vi "ODMR sweep ACCES DAC WF control.vi"(5 "leveling file":path=path "C:/Users/Ouyang Group/Documents/Data/8-26-16/Windfreak plus switches and amp power calibration high res", 6 "p (dbm)":dbl=-4.0, 7 "leveling":bool=TRUE, 8 "Save?":bool, 9 "file path (dialog if empty)":path, 10 "Freq Sweep Cluster":T1={"GPIB address 2"="19", "resolution (10 Hz:2) 2"=2, "band (1-26.5:2) 2"=2, "Freq max"=3000000000.0, "Start Freq"=2700000000.0, "Freq Step"=10000000.0, "rate"=100.0, "samples per channel"=200} {"rate" format="%0.2f"; "resolution (10 Hz:2) 2" items=["0.1 Hz", "1 Hz", "10 Hz", "100 Hz", "1 KHz", "10 KHz", "100 KHz", "1 MHz", "10 MHz", "100 MHz", "1 GHz"]}, 11 "Dot Tracking Cluster":T2={"RS232 settings"={"Portnumber"=12, "Baudrate"=5}, "X Parameters"={"Number of X Steps"=200, "Max X (V)"=2.0, "Min X (V)"=-2.0}, "Y Parameters"={"Number of Y Steps"=200, "Max Y (V)"=2.0, "Min Y (V)"=-2.0}, "X Pos"=97.0, "Y Pos"=112.0, "Z Pos"=52.78, "Tracking interval"=150.0} {"RS232 settings"."Portnumber" items=["COM1", "COM2", "COM3", "COM4", "COM5", "COM6", "COM7", "COM8", "COM9", "COM10", "COM11", "COM12", "COM13", "COM14", "COM15", "COM16", "COM17", "COM18", "COM19", "COM20", "COM21", "COM22", "COM23", "COM24", "COM25", "COM26", "COM27", "COM28", "COM29", "COM30"]; "RS232 settings"."Baudrate" items=["9600", "14400", "19200", "38400", "57600", "115200"]}) -> (0 "Z Position":dbl=31.0, 1 "Y Position":dbl=62.0, 2 "X Position":dbl=97.0, 3 "XY Graph":cluster{"Y":dbl[], "Y":dbl[]}[](graph), 4 "appended array":ext[][](array[numeric]))   [LabVIEW 2012]
uses:
  <vilib>/DAQmx/read.llb/DAQmx Read (Counter 1D DBL 1Chan NSamp).vi
  <vilib>/DAQmx/create/channels.llb/DAQmx Create Channel (CI-Count Edges).vi
  <vilib>/DAQmx/configure/timing.llb/DAQmx Timing (Sample Clock).vi
  <vilib>/DAQmx/miscellaneous.llb/DAQmx Fill In Error Info.vi
  <vilib>/Utility/file.llb/Write To Spreadsheet File (DBL).vi
  <resource>/objmgr/daqmx.rc
panel:
  out "COM Error":bool
  out "Level":bool
  out "power":dbl
  out "Frequency":dbl
  in  "stop":bool
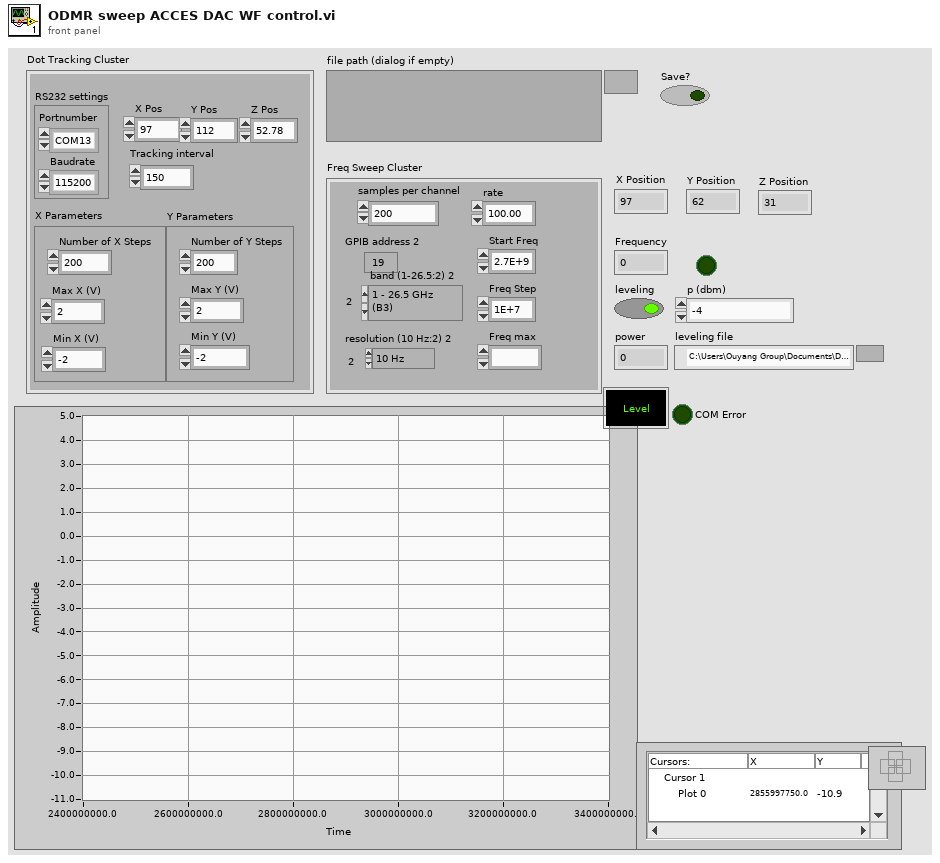
[diagram p1: front panel]
types:
  T1 = cluster{"GPIB address 2":string, "resolution (10 Hz:2) 2":i32, "band (1-26.5:2) 2":i32, "Freq max":ext, "Start Freq":dbl, "Freq Step":dbl, "rate":dbl, "samples per channel":i32}
  T2 = cluster{"RS232 settings":cluster{"Portnumber":i32, "Baudrate":u16}, "X Parameters":cluster{"Number of X Steps":i32, "Max X (V)":dbl, "Min X (V)":dbl}, "Y Parameters":cluster{"Number of Y Steps":i32, "Max Y (V)":dbl, "Min Y (V)":dbl}, "X Pos":dbl, "Y Pos":dbl, "Z Pos":dbl, "Tracking interval":dbl}
  T3 = cluster{"Number of X Steps":i32, "Max X (V)":dbl, "Min X (V)":dbl}
  T4 = cluster{"Number of Y Steps":i32, "Max Y (V)":dbl, "Min Y (V)":dbl}
  T5 = cluster{"source lock":bool, "lock frequency (Hz)":ext, "coarse tune":bool}
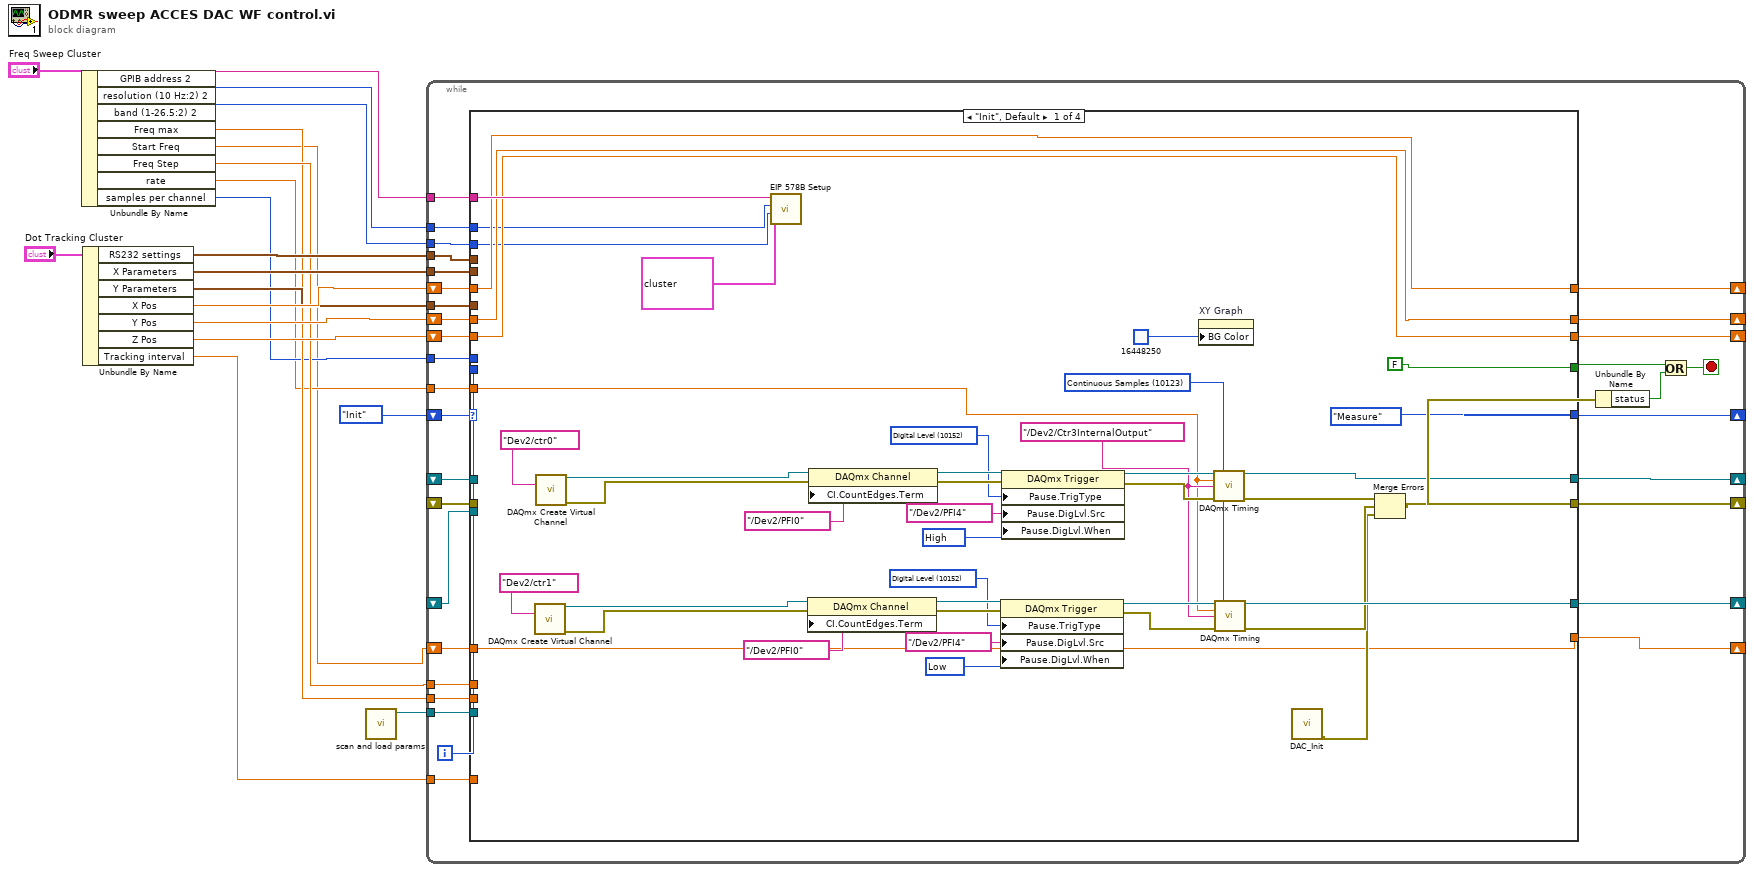
[diagram p0: block diagram]
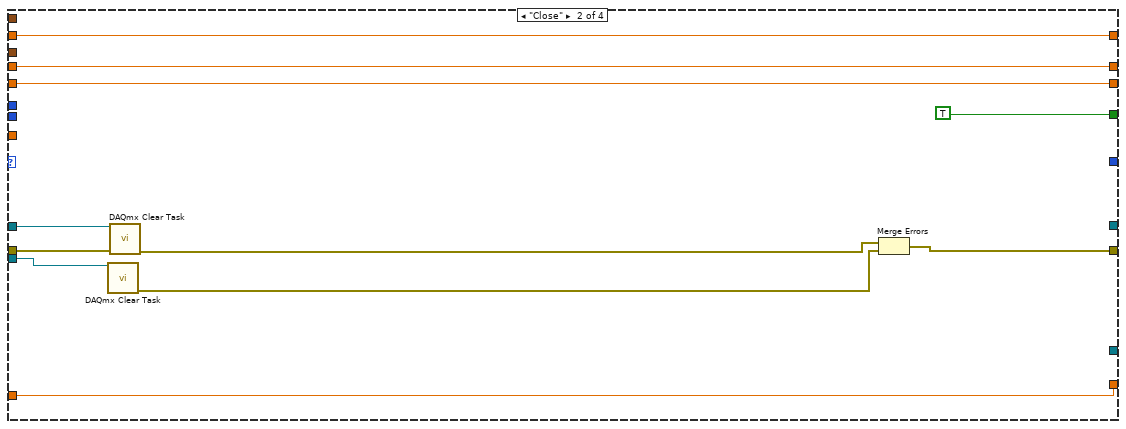
[diagram p2: hidden frame]
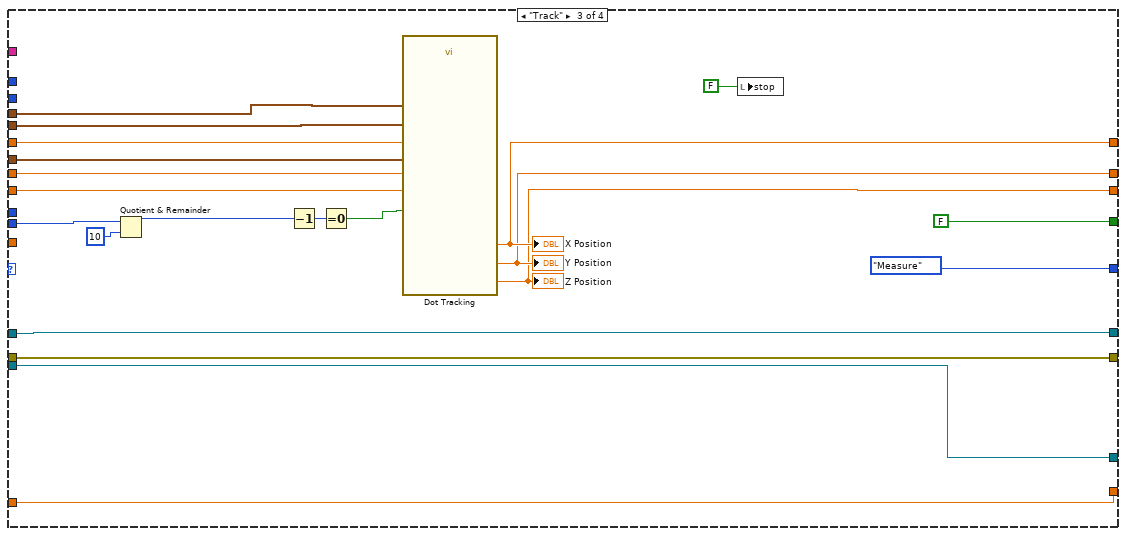
[diagram p3: hidden frame]
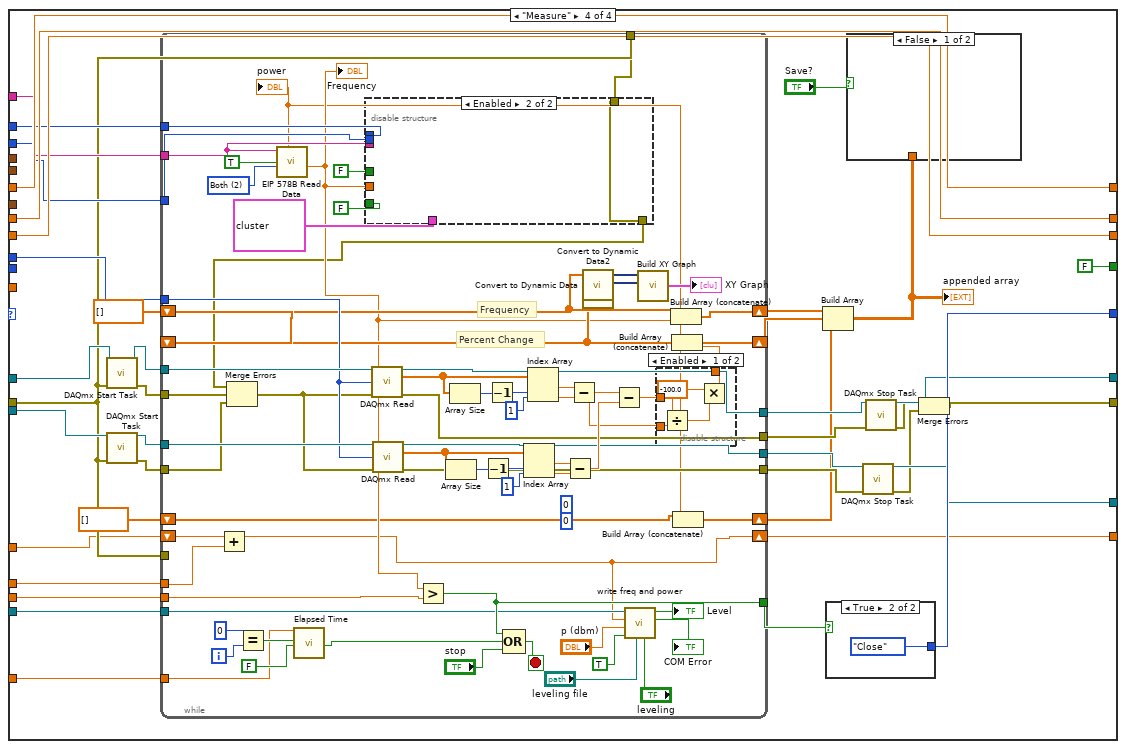
[diagram p4: hidden frame]
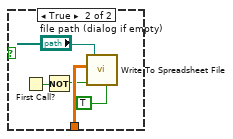
[diagram p5: hidden frame]
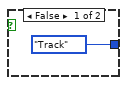
[diagram p6: hidden frame]
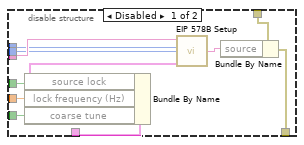
[diagram p8: hidden frame]
diagram:
  n1 = Unbundle By Name("Freq Sweep Cluster") -> ("GPIB address 2"=w9:string, "resolution (10 Hz:2) 2"=w8:i32, "band (1-26.5:2) 2"=w7:i32, "Freq max"=w5:ext, "Start Freq"=w2:dbl, "Freq Step"=w6:dbl, "rate"=w3:dbl, "samples per channel"=w4:i32)
  n2 = Unbundle By Name("Dot Tracking Cluster") -> ("RS232 settings"=w14:cluster{"Portnumber":i32, "Baudrate":u16}, "X Parameters"=w13:T3, "Y Parameters"=w12:T4, "X Pos"=w17:dbl, "Y Pos"=w16:dbl, "Z Pos"=w15:dbl, "Tracking interval"=w11:dbl)
  n3 = call "scan and load params.vi"() -> ("Serial Port Select"=w1:refnum<visa-resource-name>)  [unwired: 9 out]
  n4 = while {
    shift-right: [w47] -> _
    shift-left: enum16{"Init", "Measure", "Track", "Close"}."Init" -> [w51]
    tunnel: w9 -> [w50]
    shift-right: [w49] -> _
    shift-left: _ -> [w46]
    shift-right: [w48] -> _
    shift-left: _ -> [w45]
    shift-right: [w42] -> _
    shift-left: _ -> [w44]
    tunnel: w4 -> [w39]
    shift-right: [w34] -> _
    shift-left: w17 -> [w37]
    shift-right: [w33] -> _
    shift-left: w16 -> [w36]
    shift-right: [w32] -> _
    shift-left: w15 -> [w35]
    tunnel: w8 -> [w31]
    tunnel: w7 -> [w30]
    shift-right: [w27] -> _
    shift-left: w2 -> [w29]
    tunnel: w6 -> [w28]
    tunnel: w14 -> [w26]
    tunnel: w13 -> [w25]
    tunnel: w12 -> [w24]
    tunnel: w11 -> [w23]
    tunnel: w5 -> [w22]
    tunnel: w3 -> [w21]
    tunnel: w1 -> [w20]
    i -> [w43]
    stop <- w41 stop-if-true
    n5 = case shown="\"Init\", Default" w51 {
      tunnel: [FALSE TRUE FALSE FALSE] -> w40
      tunnel: w50 -> [w92 _ _ w142]
      tunnel: [w67 _ w125 w154] -> w49
      tunnel: [w66 _ w124 w151] -> w48
      tunnel: [w63 w99 w118 w164] -> w42
      tunnel: [enum16{"Init", "Measure", "Track", "Close"}."Measure" _ enum16{"Init", "Measure", "Track", "Close"}."Measure" w163] -> w47
      tunnel: w46 -> [_ w103 w125 w160]
      tunnel: w45 -> [_ w101 w124 w157]
      tunnel: w44 -> [_ w102 w118 w137]
      tunnel: w43 -> [_ _ w119 _]
      tunnel: w39 -> [_ _ _ w147]
      tunnel: w37 -> [w59 w97 w114 w145]
      tunnel: w36 -> [w58 w96 w113 w144]
      tunnel: w35 -> [w57 w95 w112 w143]
      tunnel: [w59 w97 w111 w145] -> w34
      tunnel: [w58 w96 w110 w144] -> w33
      tunnel: [w57 w95 w109 w143] -> w32
      tunnel: w31 -> [w56 _ _ w141]
      tunnel: w30 -> [w55 _ _ w140]
      tunnel: w29 -> [w53 w94 w108 w136]
      tunnel: w28 -> [_ _ _ w135]
      tunnel: [w53 w94 w108 w134] -> w27
      tunnel: w26 -> [_ _ w107 _]
      tunnel: w25 -> [_ _ w106 _]
      tunnel: w24 -> [_ _ w105 _]
      tunnel: w23 -> [_ _ _ w133]
      tunnel: w22 -> [_ _ _ w132]
      tunnel: w21 -> [w52 _ _ _]
      tunnel: w20 -> [_ _ _ w126]
      frame "Init", Default {
        w68 = tag "/Dev2/Ctr3InternalOutput" ("source")
        w69 = 10123 items=["Finite Samples"=10178, "Continuous Samples"=10123, "Hardware Timed Single Point"=12522] ("sample mode")
        w74 = 10214 items=["High"=10192, "Low"=10214] ("Pause.DigLvl.When")
        w76 = 10152 items=["Analog Level"=10101, "Analog Window"=10103, "Digital Level"=10152, "Digital Pattern"=10398, "None"=10230] ("Pause.TrigType")
        w83 = 10192 items=["High"=10192, "Low"=10214] ("Pause.DigLvl.When")
        w85 = 10152 items=["Analog Level"=10101, "Analog Window"=10103, "Digital Level"=10152, "Digital Pattern"=10398, "None"=10230] ("Pause.TrigType")
        n6 = call-poly <vilib>:"DAQmx Create Virtual Channel.vi"("counter"=tag "Dev2/ctr1") -> ("task out"=w81:refnum<k21>, "error out"=w80:errorcluster)  [unwired: 13 in]
        n7 = call-poly <vilib>:"DAQmx Create Virtual Channel.vi"("counter"=tag "Dev2/ctr0") -> ("task out"=w90:refnum<k21>, "error out"=w89:errorcluster)  [unwired: 13 in]
        n8 = call "EIP 578B Setup.vi"("GPIB Address"=w92, "band (1-26.5 GHz:20)"=w56, "resolution (1 Hz:1)"=w55, "source locking"=T5 {"source lock"=FALSE, "lock frequency (Hz)"=1000000000.0, "coarse tune"=TRUE}) -> ()  [unwired: 2 in, 2 out]
        n9 = property class="DAQmx Channel"(reference=w81, error in=w80, "CI.CountEdges.Term"=tag "/Dev2/PFI0") -> (reference out=w78:refnum<k21>, error out=w77:errorcluster)
        n10 = property class="DAQmx Channel"(reference=w90, error in=w89, "CI.CountEdges.Term"=tag "/Dev2/PFI0") -> (reference out=w87:refnum<k21>, error out=w86:errorcluster)
        n11 = property class="DAQmx Trigger"(reference=w78, error in=w77, "Pause.TrigType"=w76, "Pause.DigLvl.Src"=tag "/Dev2/PFI4", "Pause.DigLvl.When"=w74) -> (reference out=w71:refnum<k21>, error out=w70:errorcluster)
        n12 = property class="DAQmx Trigger"(reference=w87, error in=w86, "Pause.TrigType"=w85, "Pause.DigLvl.Src"=tag "/Dev2/PFI4", "Pause.DigLvl.When"=w83) -> (reference out=w73:refnum<k21>, error out=w72:errorcluster)
        n13 = property on="XY Graph" class="XYGraph (strict)"("BG Color"=u32 16448250) -> ()  [unwired: 2 in, 2 out]
        n14 = call-poly <vilib>:"DAQmx Timing.vi"("task/channels in"=w73, "sample mode"=w69, "rate"=w52, "source"=w68, "error in"=w72) -> ("task out"=w67:refnum<k21>, "error out"=w65:errorcluster)  [unwired: 9 in]
        n15 = call-poly <vilib>:"DAQmx Timing.vi"("task/channels in"=w71, "sample mode"=w69, "rate"=w52, "source"=w68, "error in"=w70) -> ("task out"=w66:refnum<k21>, "error out"=w64:errorcluster)  [unwired: 9 in]
        n16 = call "DAC_Init.vi"() -> ("error out"=w54:errorcluster)  [unwired: 11 in]
        n17 = Merge Errors(w65, w64, w54) -> (w63:errorcluster)
      }
      frame "Close" {
        n18 = call <vilib>:"DAQmx Clear Task.vi"("task in"=w101) -> ("error out"=w100:errorcluster)  [unwired: 14 in]
        n19 = call <vilib>:"DAQmx Clear Task.vi"("task in"=w103, "error in"=w102) -> ("error out"=w98:errorcluster)  [unwired: 13 in]
        n20 = Merge Errors(w98, w100) -> (w99:errorcluster)
      }
      frame "Track" {
        n21 = Quotient & Remainder(x=w119, y=10) -> (x-y*floor(x/y)=w122:i32)  [unwired: 1 out]
        n22 = Decrement(x=w122) -> (x-1=w123:i32)
        n23 = Equal To 0?(x=w123) -> (x = 0?=w120:bool)
        n24 = call "Dot Tracking.vi"("X"=w106, "Y Parameters"=w105, "RS232 settings"=w107, "X Pos"=w114, "Y pos"=w113, "Z Pos"=w112, "Z-track?"=w120) -> ("X Position"=w111:dbl, "Y Position"=w110:dbl, "Z Position"=w109:dbl)  [unwired: 2 in, 4 out]
        "X Position" <- w111
        "Y Position" <- w110
        "Z Position" <- w109
        n25 = local write "stop"(FALSE ("stop")) -> ()
      }
      frame "Measure" {
        w146 = dbl[] []
        n26 = call <vilib>:"DAQmx Start Task.vi"("task/channels in"=w160, "error in"=w137) -> ("task out"=w158:refnum<k21>, "error out"=w159:errorcluster)  [unwired: 12 in]
        n27 = call <vilib>:"DAQmx Start Task.vi"("task/channels in"=w157, "error in"=w137) -> ("task out"=w156:refnum<k21>, "error out"=w155:errorcluster)  [unwired: 12 in]
        n28 = while {
          shift-right: [w225] -> w149
          shift-left: w146 -> [w212]
          shift-right: [w224] -> w130
          shift-left: w146 -> [w214]
          tunnel: w156 -> [w221]
          tunnel: [w220] -> w153
          tunnel: [w219] -> w162
          tunnel: [w216] -> w161
          tunnel: w159 -> [w218]
          tunnel: w158 -> [w217]
          tunnel: w155 -> [w190]
          tunnel: w147 -> [w215]
          tunnel: w142 -> [w202]
          tunnel: w141 -> [w201]
          tunnel: w140 -> [w200]
          tunnel: w137 -> [w192]
          tunnel: [w188] -> w139
          tunnel: [w187] -> w138
          tunnel: w137 -> [_]
          shift-right: [w178] -> w134
          shift-left: w136 -> [w186]
          tunnel: w135 -> [w185]
          tunnel: w133 -> [w184]
          tunnel: w132 -> [w183]
          shift-right: [w182] -> w127
          shift-left: dbl[] [] -> [w181]
          tunnel: w126 -> [w179]
          i -> [w204]
          stop <- w193 stop-if-true
          (unwired) u16 0 ("Channel")
          (unwired) u64 0 ("DeviceIndex")
          w208 = 2 items=["Frequency", "Power", "Both"] ("output mode (freq:0)")
          # "Percent Change"
          # "Frequency"
          n29 = Add(x=w186, y=w185) -> (x+y=w178:dbl)
          n30 = Equal?(x=0, y=w204) -> (x = y?=w203:bool)
          n31 = call "EIP 578B Read Data.vi"("output mode (freq:0)"=w208, "fast (T=active)"=TRUE, "GPIB"=w202) -> ("Power (dBm)"=w180:ext, "frequency (Hz)"=w196:ext)  [unwired: 1 in, 2 out]
          "Frequency" <- w196
          "power" <- w180
          n32 = call "Elapsed Time"("Time Target (s)"=w184, "Reset"=w203, "Auto Reset"=FALSE) -> ("Time has Elapsed"=w195:bool)  [unwired: 9 in, 7 out]
          n33 = disable-structure shown="Enabled" {
            disable-tunnel: w202 -> [w255 _]
            disable-tunnel: w201 -> [w254 _]
            disable-tunnel: w200 -> [w253 _]
            disable-tunnel: T5 {"source lock"=FALSE, "lock frequency (Hz)"=1000000000.0, "coarse tune"=TRUE} ("source locking") -> [w252 _]
            disable-tunnel: FALSE ("source lock") -> [w251 _]
            disable-tunnel: FALSE ("coarse tune") -> [w250 _]
            disable-tunnel: w196 -> [w248 _]
            disable-tunnel: w192 -> [w247 w256]
            disable-tunnel: [w245 w256] -> w191
            frame Disabled {
              n34 = Bundle By Name(cluster=w252, "source lock"=w251, "lock frequency (Hz)"=w248, "coarse tune"=w250) -> (w249:T5)
              n35 = call "EIP 578B Setup.vi"("GPIB Address"=w255, "band (1-26.5 GHz:20)"=w254, "resolution (1 Hz:1)"=w253, "source locking"=w249) -> ("status messages"=w246:string)  [unwired: 2 in, 1 out]
              n36 = Bundle By Name(cluster=w247, "source"=w246) -> (w245:errorcluster)
            }
            frame Enabled {
            }
          }
          n37 = Merge Errors(w191, w218, w190) -> (w189:errorcluster)
          n38 = call-poly <vilib>:"DAQmx Read.vi"("task/channels in"=w217, "number of samples per channel"=w215, "error in"=w189) -> ("task out"=w219:refnum<k21>, "data"=w238:dbl[], "error out"=w220:errorcluster)  [unwired: 10 in]
          n39 = call-poly <vilib>:"DAQmx Read.vi"("task/channels in"=w221, "number of samples per channel"=w215, "error in"=w189) -> ("task out"=w216:refnum<k21>, "data"=w227:dbl[], "error out"=w187:errorcluster)  [unwired: 10 in]
          n40 = Greater?(x=w196, y=w183) -> (0:w188:bool)
          n41 = Array Size(array=w227) -> (size(s)=w232:i32)
          n42 = Array Size(array=w238) -> (size(s)=w237:i32)
          n43 = Decrement(x=w232) -> (x-1=w231:i32)
          n44 = Decrement(x=w237) -> (x-1=w236:i32)
          n45 = Compound Arithmetic op=OR(w188, w195, "stop") -> (w193:bool)
          n46 = Index Array(array=w227, index #1=w231, index #2=1 ("index")) -> (element #1=w228:dbl, element #2=w229:dbl)
          n47 = Index Array(array=w238, index #1=w236, index #2=1 ("index")) -> (element #1=w233:dbl, element #2=w234:dbl)
          n48 = Subtract(x=w228, y=w229) -> (x-y=w226:dbl)
          n49 = Subtract(x=w233, y=w234) -> (x-y=w222:dbl)
          n50 = call "Convert to Dynamic Data"("Array"=w214) -> ("Dynamic Data Type"=w213:dynamicdata)  [unwired: 3 in]
          n51 = call "Convert to Dynamic Data2"("Array"=w212) -> ("Dynamic Data Type"=w211:dynamicdata)  [unwired: 3 in]
          n52 = Subtract(x=w222, y=w226) -> (x-y=w223:dbl)
          n53 = call "write freq and power.vi"("leveling"="leveling", "leviling file"="leveling file", "RF On"=TRUE, "p (dbm)"="p (dbm)", "f (Hz)"=w178, "Serial Port Select"=w179) -> ("COM Error"=→"COM Error":bool, "Level"=→"Level":bool)  [unwired: 4 in]
          n54 = call "Build XY Graph"("Y Input"=w211, "X Input"=w213) -> ("XY Graph"=→"XY Graph":cluster{"Y":dbl[], "Y":dbl[]}[])  [unwired: 3 in, 6 out]
          n55 = disable-structure shown="Enabled" {
            disable-tunnel: w223 -> [w243 w244]
            disable-tunnel: w222 -> [w242 _]
            disable-tunnel: [w240 w244] -> w209
            frame Enabled {
              n56 = Divide(x=w243, y=w242) -> (x/y=w241:dbl)
              n57 = Multiply(x=-100.0, y=w241) -> (x*y=w240:dbl)
            }
            frame Disabled {
            }
          }
          n58 = Build Array (concatenate)(w214, w196) -> (w224:ext[])
          n59 = Build Array (concatenate)(w212, w209) -> (w225:dbl[])
          n60 = Build Array (concatenate)(w181, w180) -> (w182:ext[])
        }
        n61 = Build Array(w130, w149, w127) -> (w148:ext[][])
        "appended array" <- w148
        n62 = case shown="True" w139 {
          tunnel: [enum16{"Init", "Measure", "Track", "Close"}."Track" enum16{"Init", "Measure", "Track", "Close"}."Close"] -> w163
          frame False {
          }
          frame True {
          }
        }
        n63 = case shown="False" "Save?" {
          tunnel: w148 -> [_ w169]
          frame False {
          }
          frame True {
            n64 = First Call?() -> (First Call?: T/F=w168:bool)
            n65 = Not(x=w168) -> (.not. x?=w167:bool)
            n66 = call-poly <vilib>:"Write To Spreadsheet File.vi"("transpose? (no:F)"=TRUE, "append to file? (new file:F)"=w167, "2D data"=w169, "file path (dialog if empty)"="file path (dialog if empty)") -> ()  [unwired: 4 in, 1 out]
          }
        }
        n67 = call <vilib>:"DAQmx Stop Task.vi"("task/channels in"=w161, "error in"=w138) -> ("task out"=w151:refnum<k21>, "error out"=w150:errorcluster)  [unwired: 12 in]
        n68 = call <vilib>:"DAQmx Stop Task.vi"("task/channels in"=w162, "error in"=w153) -> ("task out"=w154:refnum<k21>, "error out"=w152:errorcluster)  [unwired: 12 in]
        n69 = Merge Errors(w152, w150) -> (w164:errorcluster)
      }
    }
    n70 = Unbundle By Name(w42) -> ("status"=w38:bool)
    n71 = Or(x=w40, y=w38) -> (x .or. y?=w41:bool)
  }
